vi "WriteTextFiles.vi"(1 "error in":errorcluster, 2 "Action #":i32, 3 "RT Actions":T1 {"Slow AO Array"."Duration, Gain, NewVal" format="%#_3g"}, 4 "Txt cmds":string[](array[string])) -> (0 "error out":errorcluster)   [LabVIEW 2018]
uses:
  RT Actions.ctl
  RT/ActionCluster.ctl
  RT/Instructions_RT.ctl
  RT/ParameterSubCluster.ctl
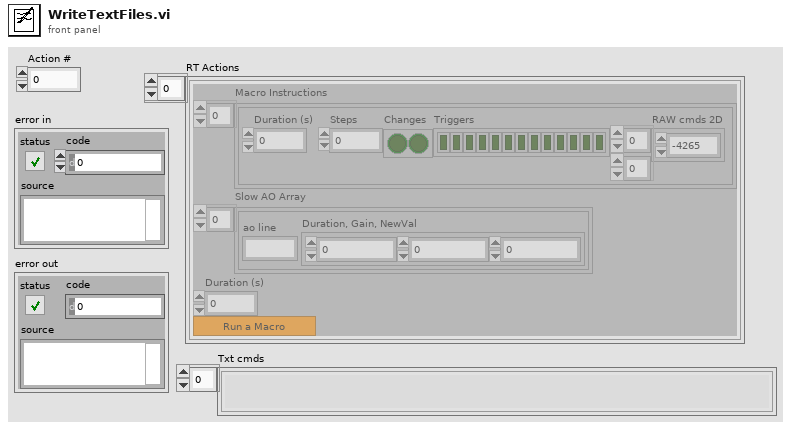
[diagram p1: front panel]
types:
  T1 = typedef "RT Actions.ctl" = T2[]
  T2 = typedef "ActionCluster.ctl" = cluster{"Macro Instructions":T3, "Slow AO Array":T4, "Duration (s)":dbl, "Toggle":bool}
  T3 = typedef "Instructions_RT.ctl" = cluster{"Duration (s)":dbl, "Steps":i32, "Changes":bool[], "Triggers":bool[], "RAW cmds 2D":i16[][]}[]
  T4 = typedef "ParameterSubCluster.ctl" = cluster{"ao line":string, "Duration, Gain, NewVal":dbl[]}[]
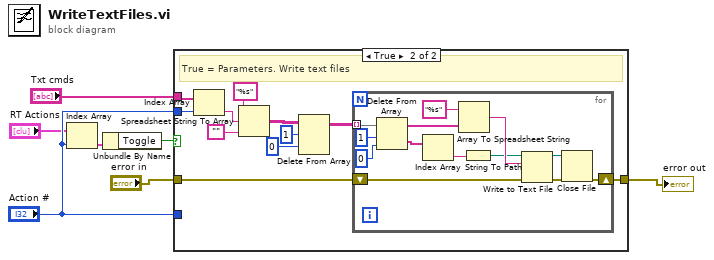
[diagram p0: block diagram]
diagram:
  n1 = Index Array(array="RT Actions", index="Action #") -> (element=w5:T2)
  n2 = Unbundle By Name(w5) -> ("Toggle"=w3:bool)
  n3 = case shown="True" w3 {
    tunnel: "Action #" -> [_ _]
    tunnel: "Txt cmds" -> [_ w19]
    tunnel: "Action #" -> [_ w18]
    tunnel: "error in" -> [w8 w11]
    tunnel: [w8 w10] -> w1
    frame False {
      # "False = Macro. Do nothing"
    }
    frame True {
      # "True = Parameters. Write text files"
      n4 = Index Array(array=w19, index=w18) -> (element=w16:string)
      n5 = Spreadsheet String To Array(format string="%s", spreadsheet string=w16, array type (2D Dbl)="") -> (array=w14:string[][])  [unwired: 1 in]
      n6 = Delete From Array(array=w14, length=1, index (row)=0) -> (array with subset deleted=w12:string[][])  [unwired: 1 in, 1 out]
      n7 = for {
        tunnel: w12 -> [w32] mode=indexing
        shift-right: [w24] -> w10
        shift-left: w11 -> [w20]
        n8 = Delete From Array(array=w32, length=1, index=0) -> (deleted portion=w30:string[], array with subset deleted=w29:string[])
        n9 = Index Array(array=w30) -> (element=w22:string)  [unwired: 1 in]
        n10 = Array To Spreadsheet String(array=w29, 3:"%s" ("format string")) -> (spreadsheet string=w28:string)  [unwired: 1 in]
        n11 = String To Path(string=w22) -> (path=w21:path)
        n12 = Write to Text File(file (use dialog)=w21, text=w28, error in=w20) -> (refnum out=w25:refnum<file>, error out=w26:errorcluster)  [unwired: 1 in, 1 out]
        n13 = Close File(refnum=w25, error in=w26) -> (error out=w24:errorcluster)  [unwired: 1 out]
      }
    }
  }
  "error out" <- w1
